vi "MixingGUI.vi"() -> ()   [LabVIEW 2016]
uses:
  <vilib>/Utility/miscctls.llb/LVStringsAndValuesArrayTypeDef.ctl
  <userlib>/Fluigent/Fluigent MFCS/FluigentMFCS_Full.llb/MFCS_EZ Detect.vi
  <userlib>/Fluigent/Fluigent MFCS/FluigentMFCS_Full.llb/MFCS_EZ Initialization.vi
  Labjack/ValveGlobals.vi
  Globals/PressuresGlobal.vi
  <vilib>/Utility/file.llb/Write Delimited Spreadsheet (string).vi
  <vilib>/Utility/file.llb/Read Delimited Spreadsheet (string).vi
  <userlib>/Fluigent/Fluigent MFCS/FluigentMFCS_Full.llb/MFCS_EZ Write Channel Pressure.vi
  <userlib>/_OpenG.lib/array/array.llb/Remove Duplicates from 1D Array (U16)__ogtk.vi
  <userlib>/Fluigent/Fluigent MFCS/FluigentMFCS_Full.llb/MFCS_EZ Close.vi
  <vilib>/MakerHub/Toolbox/LMH-Toolbox.lvlib
panel:
  out "Calibration Refs":T1
  out "Master Pressure Groups":u8[](array[numeric])=[3, 3, 3, 3, 4, 4, 4, 4, 2, 2]
  in  "Master Valves":u16(ring) items=["A1", "A2", "A3", "A4", "B1", "B2", "B3", "B4", "B5", "B6", "B7", "B8", "A5"]
  out "Set Pressures":dbl[][](array[numeric])
  out "Ctr Pressure":dbl=292.8560256927093
  in  "stop":bool
  in  "Tab Control":enum32{"Page 1", "Page 2"}(tab)
  in  "Reset All Calibrations":bool
  in  "Save Odor Inf File":bool
  in  "_run":i16=101
  in  "Sync Camera Acquisition":bool=TRUE
  in  "Ctr Water Valve":u16(ring)=15 items=["A1", "A2", "A3", "A4", "B1", "B2", "B3", "B4", "B5", "B6", "B7", "B8", "A5", "A6", "A7", "A8"]
  in  "Begin Experiment":bool
  in  "Log File Name":path=path "E:/maggot images/Orco_GCaMP"
  in  "Set to default pressure":bool
  in  "Mix Water Valve":u16(ring)=12 items=["A1", "A2", "A3", "A4", "B1", "B2", "B3", "B4", "B5", "B6", "B7", "B8", "A5", "A6", "A7", "A8"]
  in  "Mix Cluster":T2={"Ratio"=[0.6, 0.5], "Mix 2"=[12, 9], "Mix 1"=[0, 1]} {"Mix 1" items=["A1"=0, "A2"=1, "A3"=2, "A4"=3, "A5"=12]; "Mix 2" items=["B5"=8, "B6"=9, "B7"=10, "B8"=11, "A5"=12]}
  out "Ctr Pressure Group":u8=1
  out "Water Mix Pressure Group":u8=2
  in  "Close All Valves":bool
  in  "Odor":u16[](array[ring])=[0, 0, 0, 0, 0, 0, 0, 0] items=["1-pentanol", "3-pentanol", "3-octanol", "2,5-dimethylthiazole", "Add new..."]
  in  "Concentration":u16[](array[ring])=[0, 0, 0, 0, 0, 0, 0, 1] items=["10^-5", "10^-6", "Add new..."]
  in  "Odor Inf Path":path=path "C:/Users/Public/Documents/National Instruments/Fluigent/OdorInf/Data/OdorInfFiles/JB_20171127.txt"
  in  "Append Changes To Odor Inf File":bool=TRUE
  in  "Valves":u16[](array[ring])=[0, 1, 2, 3, 8, 9, 10, 11] items=["A1", "A2", "A3", "A4", "B1", "B2", "B3", "B4", "B5", "B6", "B7", "B8"]
  out "Pressure Group":u8[](array[numeric])=[3, 3, 3, 3, 4, 4, 4, 4]
  in  "Odor Time":dbl[](array[numeric])=[10.0, 10.0]
  in  "Water Time":dbl[](array[numeric])=[10.0, 10.0]
  in  "Number of Periods":dbl=2.0
  in  "Start Water":dbl=6.0
  out "Experiment Time (Sec)":dbl=46.0
  in  "Calibrate Pressures":bool
  out "Duplicates!":bool
  in  "Zero Pressure":bool
  in  "Ctr Odor Valve":u16(ring)=14 items=["A1", "A2", "A3", "A4", "B1", "B2", "B3", "B4", "B5", "B6", "B7", "B8", "A5", "A6", "A7", "A8"]
  in  "Calibration Mode":T3(ring)=enum."Odors Only"
  out "Calibration Required":bool=TRUE
  in  "Refill!":bool[](array[boolean])=[FALSE, FALSE, FALSE, FALSE, FALSE, FALSE, FALSE, FALSE, FALSE, FALSE, FALSE]
  out "Odor \nLevel":T4={"Tank"=10.0, "Tank 2"=10.0, "Tank 3"=10.0, "Tank 4"=10.0, "Tank 5"=10.0, "Tank 6"=10.0, "Tank 7"=10.0, "Tank 8"=10.0, "Tank 9"=10.0, "Tank 10"=10.0, "Tank 11"=10.0} {"Tank 11" scale=0.0..10.0; "Tank 10" scale=0.0..10.0; "Tank 9" scale=0.0..10.0; "Tank 8" scale=0.0..10.0; "Tank 7" scale=0.0..10.0; "Tank 6" scale=0.0..10.0; "Tank 5" scale=0.0..10.0; "Tank 4" scale=0.0..10.0; "Tank 3" scale=0.0..10.0; "Tank 2" scale=0.0..10.0; "Tank" scale=0.0..10.0}
  in  "Mix Water Pressure Channel":u16=2
  in  "Control Pressure Channel":u16=1
  out "Current Pressure":dbl[](array[numeric])=[1.2623618841171265, 1.893542766571045, 0.0, 2.524723768234253]
  in  "Manual Set Pressures":dbl[](array[numeric])=[292.8560256927093, 929.8857946603396, 888.3091798855597, 854.075528379124]
  in  "Total Odor Flow":dbl=425.0
  in  "Total Flow Setpoint":dbl=531.25
  out "Flow Meter 1 (water flow)":cluster{"[0]":dbl, "[1]":dbl}(graph)={"[0]"=0.1724137931034483, "[1]"=0.0}
  out "Flow Meter 2 (total flow)":cluster{"[0]":dbl, "[1]":dbl}(graph)={"[0]"=0.1724137931034483, "[1]"=0.0}
  in  "Values to Display":dbl=400.0
  out "Default Pressures":dbl[](array[numeric])=[292.8560256927093, 929.8857946603396, 888.3091798855597, 854.075528379124]
  in  "Master Ratio":dbl[](array[numeric])=[0.6, 0.6]
  in  "Master Mix 2":u16[](array[ring])=[12, 9, 11, 12, 11, 4, 4, 4] items=["B1"=4, "B2"=5, "B3"=6, "B4"=7, "A5"=12]
  in  "Master Mix 1":u16[](array[ring])=[0, 1, 1, 0, 0, 0, 0, 0] items=["A1"=0, "A2"=1, "A3"=2, "A4"=3, "A5"=12]
  in  "Master Water Time":dbl[](array[numeric])=[10.0, 10.0, 10.0, 10.0, 10.0, 10.0, 10.0, 10.0]
  in  "Master Odor Time":dbl[](array[numeric])=[10.0, 10.0, 10.0, 10.0, 10.0, 10.0, 10.0, 10.0]
  out "A5 in Both!":bool
  out "Master Valves":T5=[{"String"="A1", "Value"=0.0}, {"String"="A2", "Value"=1.0}, {"String"="A3", "Value"=2.0}, {"String"="A4", "Value"=3.0}, {"String"="B1", "Value"=4.0}, {"String"="B2", "Value"=5.0}, {"String"="B3", "Value"=6.0}, {"String"="B4", "Value"=7.0}, {"String"="B5", "Value"=8.0}, {"String"="B6", "Value"=9.0}, {"String"="B7", "Value"=10.0}, {"String"="B8", "Value"=11.0}, {"String"="A5", "Value"=12.0}]
  # "log_"
  # ".txt"
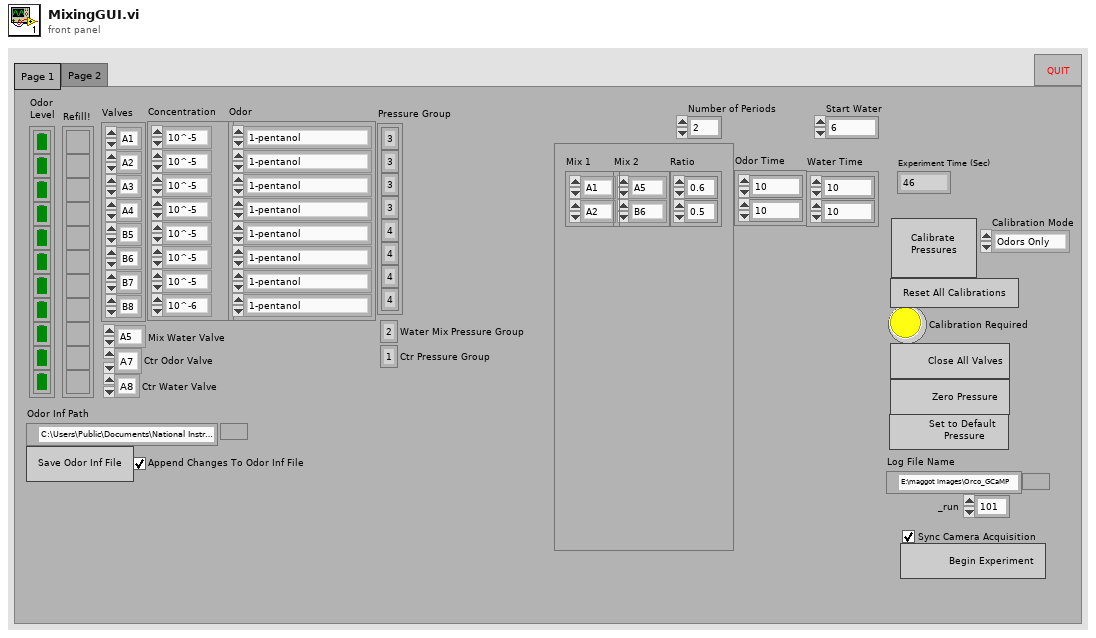
[diagram p1: front panel]
types:
  T1 = cluster{"Pressure Controller List":u8[], "Ratio List":dbl[], "Valve List":u16[]}
  T2 = cluster{"Ratio":dbl[], "Mix 2":u16[], "Mix 1":u16[]}
  T3 = enum16{"Calibrate All", "Control Only", "Odors Only"}
  T4 = cluster{"Tank":dbl, "Tank 2":dbl, "Tank 3":dbl, "Tank 4":dbl, "Tank 5":dbl, "Tank 6":dbl, "Tank 7":dbl, "Tank 8":dbl, "Tank 9":dbl, "Tank 10":dbl, "Tank 11":dbl}
  T5 = typedef "LVStringsAndValuesArrayTypeDef.ctl" = cluster{"String":string, "Value":ext}[]
  T6 = enum32{"Invalid", "Standard", "Closed", "Hidden", "Minimized", "Maximized"}
  T7 = cluster{"Ctr Odor Valve":u16, "Water Mix Valve":u16, "Total Odor Flow":dbl, "Total Flow Setpoint":dbl, "Control Pressure Channel":u16, "Mix Water Pressure Channel":u16}
  T8 = enum32{"Invalid", "Standard", "Closed", "Hidden", "Minimized", "Maximized"}[]
  T9 = typedef "_EZmfcsSN.ctl" = u16
  T10 = typedef "_EZmfcsRefNum.ctl" = refnum<k1>
  T11 = cluster{"[0]":dbl, "[1]":dbl, "[2]":dbl, "[3]":dbl, "[4]":dbl, "[5]":dbl, "[6]":dbl, "[7]":dbl, "[8]":dbl, "[9]":dbl, "[10]":dbl}
  T12 = cluster{"Flowboards":enum16{"A", "B", "C"}[], "Channels":enum16{"1", "2", "3", "4", "5", "6", "7", "8"}[], "States":bool[]}[]
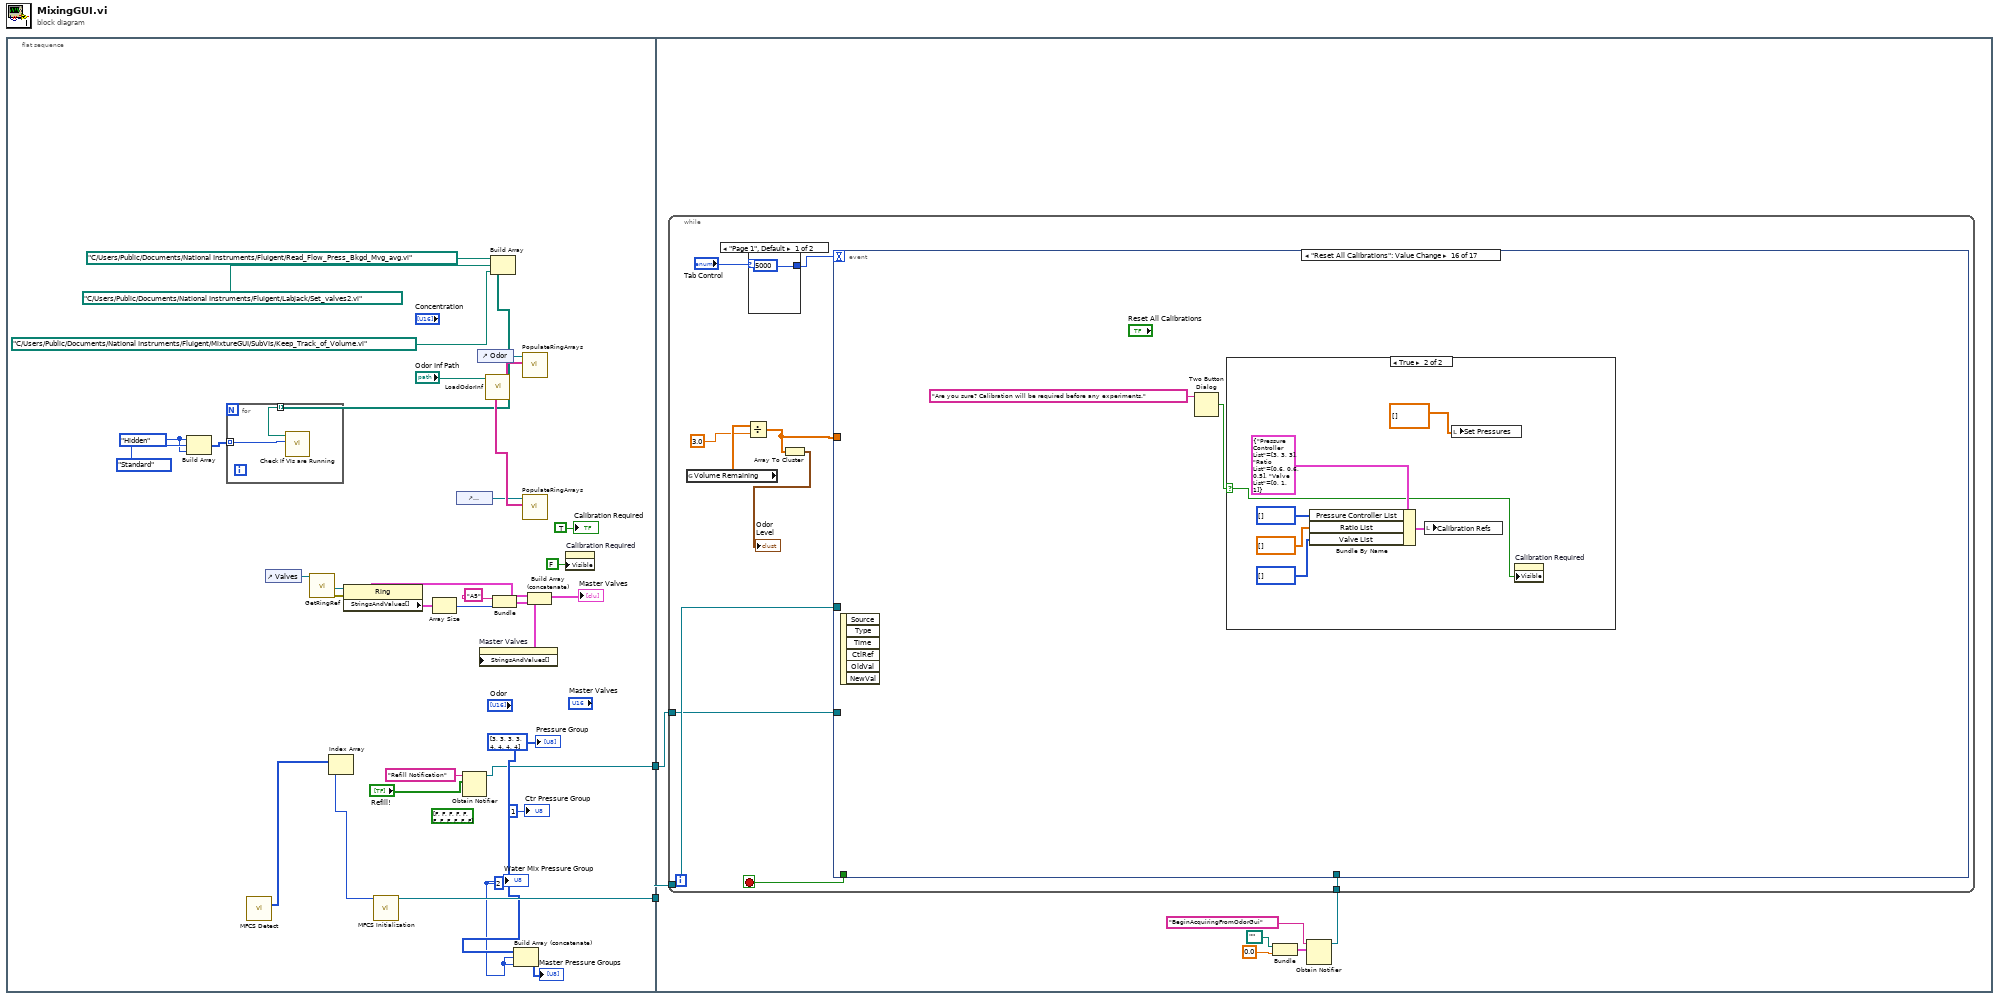
[diagram p0: block diagram]
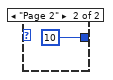
[diagram p2: hidden frame]
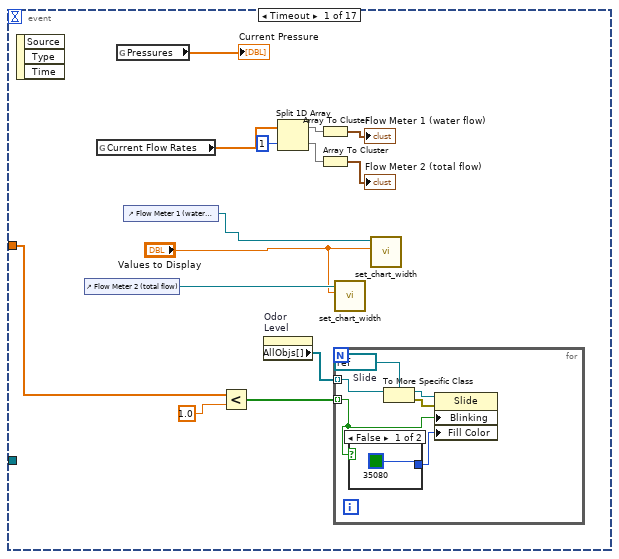
[diagram p3: hidden frame]
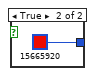
[diagram p4: hidden frame]
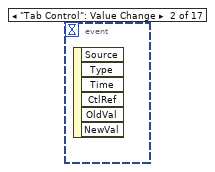
[diagram p5: hidden frame]
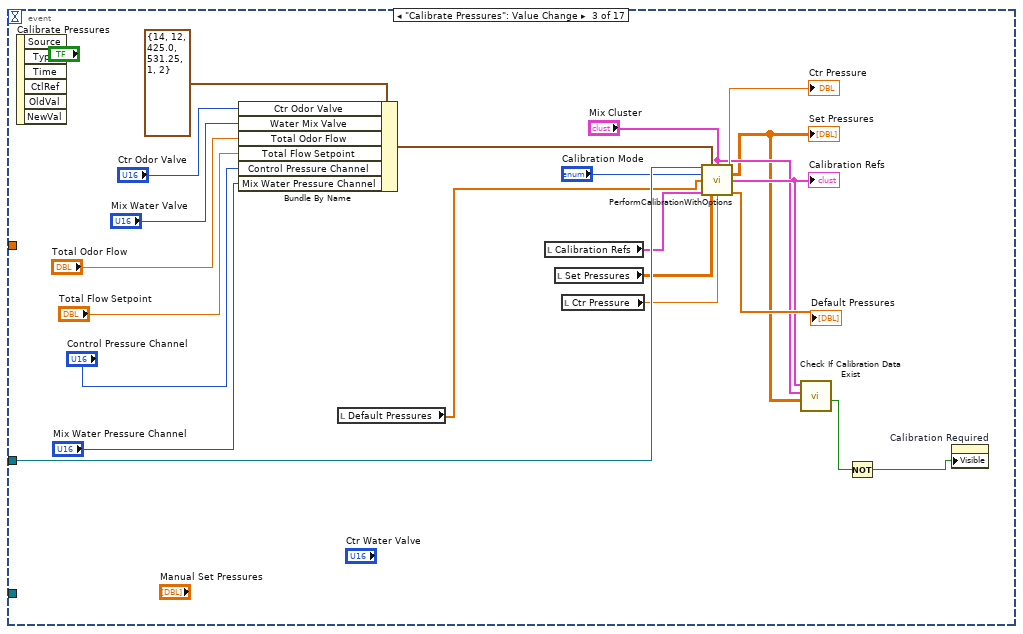
[diagram p6: hidden frame]
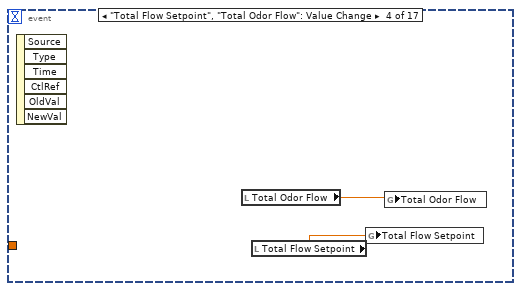
[diagram p7: hidden frame]
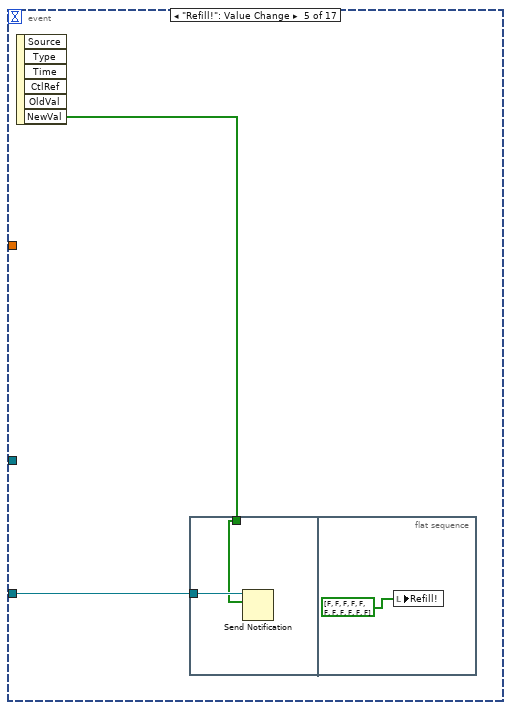
[diagram p8: hidden frame]
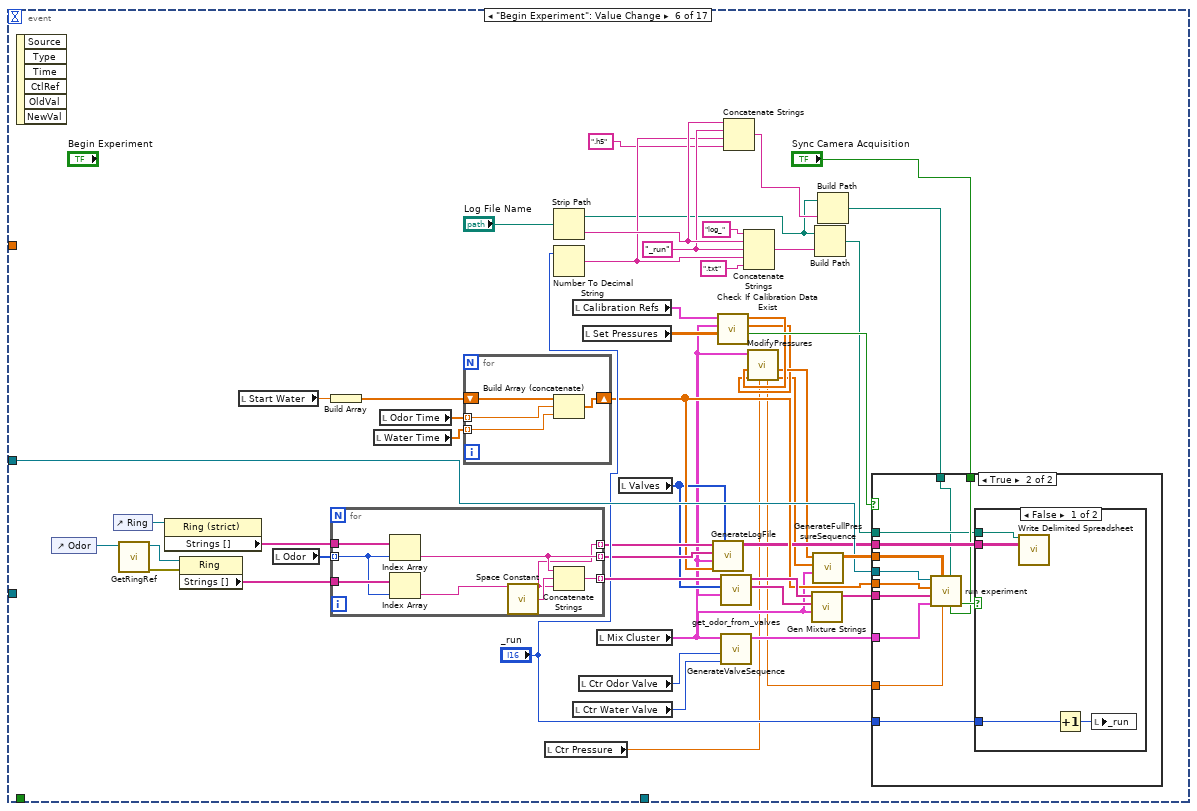
[diagram p9: hidden frame]
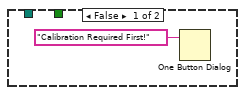
[diagram p10: hidden frame]
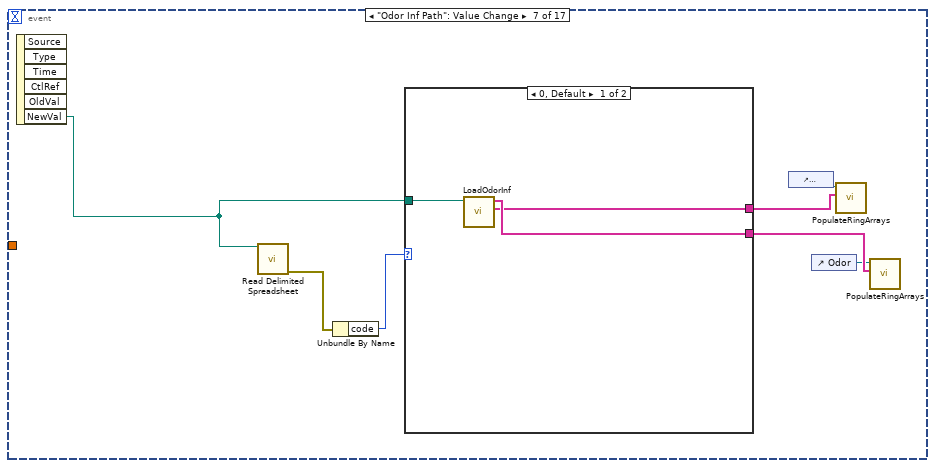
[diagram p12: hidden frame]
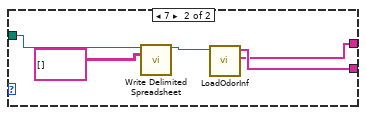
[diagram p13: hidden frame]
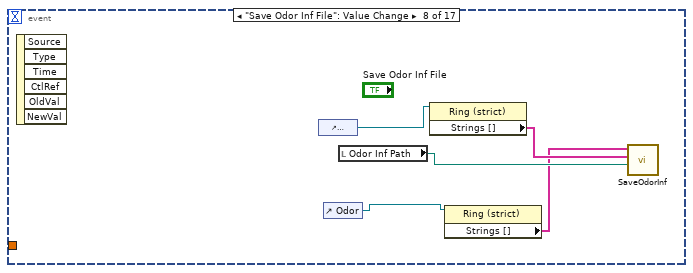
[diagram p14: hidden frame]
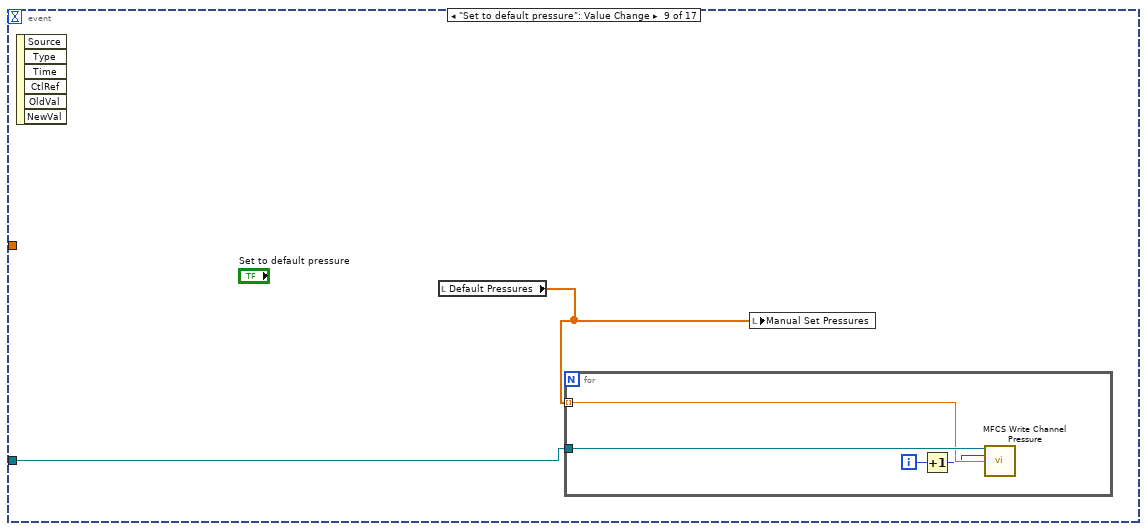
[diagram p15: hidden frame]
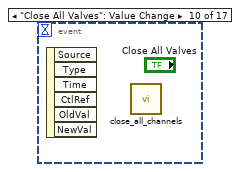
[diagram p16: hidden frame]
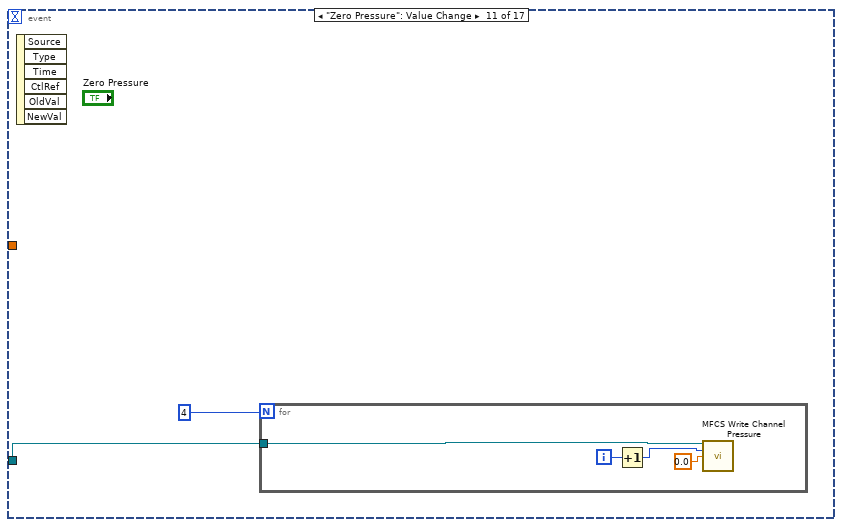
[diagram p17: hidden frame]
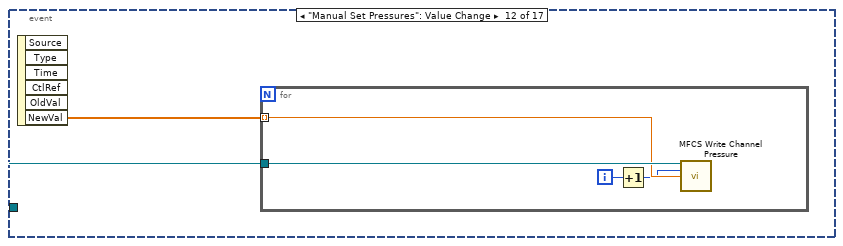
[diagram p18: hidden frame]
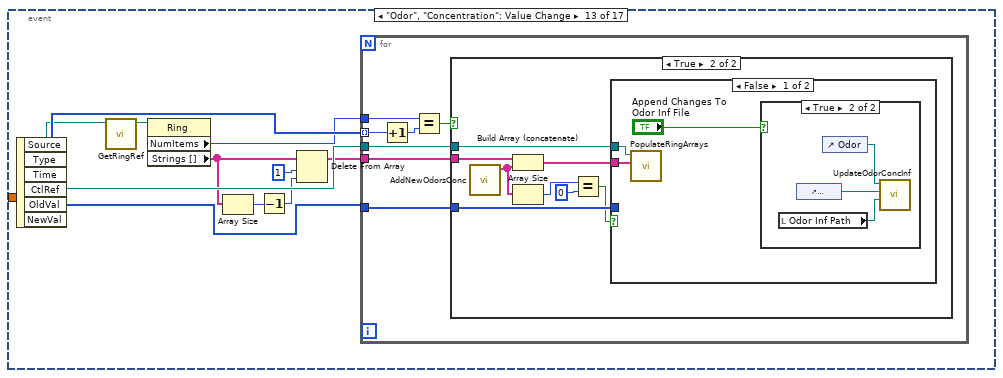
[diagram p19: hidden frame]
diagram:
  n1 = flat-sequence {
    tunnel: [w20] -> w2
    tunnel: [w6] -> w1
    tunnel: w2 -> [w43]
    tunnel: w1 -> [w37]
    frame #0 {
      (unwired) bool[] [FALSE, FALSE, FALSE, FALSE, FALSE, FALSE, FALSE, FALSE, FALSE, FALSE, FALSE] ("Refill!")
      w4 = T6."Hidden" ("State")
      w16 = u8 2 ("Water Mix Pressure Group")
      w18 = u8[] [3, 3, 3, 3, 4, 4, 4, 4] ("Pressure Group")
      n2 = Build Array(w4, T6."Standard" ("State"), w4) -> (w10:T8)
      n3 = call-poly <userlib>:"MFCS Detect.vi"() -> ("[SN MFCS_EZ]"=w22:T9[])  [unwired: 14 in, 1 out]
      n4 = control-ref of="Valves"() -> (w30:refnum<vi>)
      n5 = call "GetRingRef.vi"("Array Reference"=w30) -> ("error out"=w29:errorcluster, "Ring Reference"=w28:refnum<vi>)  [unwired: 9 in]
      n6 = Index Array(array=w22) -> (element=w21:T9)  [unwired: 1 in]
      n7 = property class="Ring"(reference=w28, error in=w29) -> ("StringsAndValues[]"=w34:T5)  [unwired: 2 out]
      n8 = call-poly <userlib>:"MFCS Initialization.vi"("SN MFCS_EZ"=w21) -> ("MFCS_EZ"=w20:T10)  [unwired: 12 in, 2 out]
      n9 = Array Size(array=w34) -> (size(s)=w32:i32)
      n10 = control-ref of="Concentration"() -> (w26:refnum<vi>)
      n11 = Obtain Notifier(name (unnamed)="Refill Notification", notification data type="Refill!") -> (notifier out=w6:refnum<notifier>)  [unwired: 2 in, 2 out]
      n12 = control-ref of="Odor"() -> (w24:refnum<vi>)
      n13 = call "LoadOdorInf.vi"("file path (dialog if empty)"="Odor Inf Path") -> ("Concentration"=w27:string[], "Odor"=w25:string[])  [unwired: 9 in]
      n14 = Build Array(path "C:/Users/Public/Documents/National Instruments/Fluigent/Read_Flow_Press_Bkgd_Mvg_avg.vi", path "C:/Users/Public/Documents/National Instruments/Fluigent/Labjack/Set_valves2.vi", path "C:/Users/Public/Documents/National Instruments/Fluigent/MixtureGUI/SubVIs/Keep_Track_of_Volume.vi") -> (w12:path[])
      n15 = for {
        tunnel: w12 -> [w36] mode=indexing
        tunnel: w10 -> [w35] mode=indexing
        n16 = call "Check If VIs are Running.vi"("State"=w35, "Path"=w36) -> ()  [unwired: 9 in, 1 out]
      }
      n17 = Bundle("A5", w32) -> (w33:cluster{string, i32})  [unwired: 1 in]
      n18 = Build Array (concatenate)(w18, w16, w16) -> (→"Master Pressure Groups":u8[])
      n19 = call "PopulateRingArrays.vi"("array"=w25, "Array Reference"=w24) -> ()  [unwired: 8 in, 2 out]
      n20 = call "PopulateRingArrays.vi"("array"=w27, "Array Reference"=w26) -> ()  [unwired: 8 in, 2 out]
      n21 = Build Array (concatenate)(w34, w33) -> (w19:T5)
      "Master Valves" <- w19
      n22 = property on="Master Valves" class="Ring (strict)"("StringsAndValues[]"=w19) -> ()  [unwired: 2 in, 2 out]
      n23 = property on="Calibration Required" class="Bool (strict)"("Visible"=FALSE) -> ()  [unwired: 2 in, 2 out]
      "Pressure Group" <- w18
      "Water Mix Pressure Group" <- w16
      "Ctr Pressure Group" <- u8 1 ("Ctr Pressure Group")
      "Calibration Required" <- TRUE ("Calibration Required")
    }
    frame #1 {
      n24 = Bundle("Log File Name"=path "", 0.0) -> (w39:cluster{"Log File Name":path, dbl})  [unwired: 1 in]
      n25 = Obtain Notifier(name (unnamed)="BeginAcquiringFromOdorGui", notification data type=w39) -> (notifier out=w41:refnum<notifier>)  [unwired: 2 in, 2 out]
      n26 = while {
        tunnel: w43 -> [w50]
        tunnel: w41 -> [w49]
        tunnel: w37 -> [w48]
        stop <- w53 stop-if-true
        n27 = global read "ValveGlobals.vi" "Volume Remaining"() -> (w47:dbl[])
        n28 = Divide(x=w47, y=3.0) -> (x/y=w44:dbl[])
        n29 = case shown="\"Page 1\", Default" "Tab Control" {
          tunnel: [5000 10] -> w51
          frame "Page 1", Default {
          }
          frame "Page 2" {
          }
        }
        n30 = Array To Cluster(array=w44) -> (cluster=→"Odor \nLevel":T11)
        n31 = event shown="[15] \"Reset All Calibrations\": Value Change" {
          selector: _ -> [_ _ _ _ _ _ _ _ _ _ _ _ _ _ _ _ _]
          dyn-events: _ -> [_ _ _ _ _ _ _ _ _ _ _ _ _ _ _ _ _]
          timeout: w51 -> [_ _ _ _ _ _ _ _ _ _ _ _ _ _ _ _ _]
          tunnel: [_ _ _ _ _ _ _ _ _ _ _ _ _ _ _ _ TRUE] -> w53
          tunnel: w50 -> [_ _ w98 _ _ w134 _ _ w203 _ w209 w216 _ _ _ _ w365]
          tunnel: w49 -> [_ _ _ _ _ _ _ _ _ _ _ _ _ _ _ _ _]
          tunnel: w48 -> [_ _ _ _ w102 _ _ _ _ _ _ _ _ _ _ _ _]
          tunnel: w44 -> [w56 _ _ _ _ _ _ _ _ _ _ _ _ _ _ _ _]
          event Timeout {
            n32 = event-data() -> ()  [unwired: 1 in, 3 out]
            n33 = control-ref of="Flow Meter 2 (total flow)"() -> (w61:refnum<vi>)
            n34 = global read "PressuresGlobal.vi" "Current Flow Rates"() -> (w66:dbl[])
            n35 = global read "PressuresGlobal.vi" "Pressures"() -> (→"Current Pressure":dbl[])
            n36 = control-ref of="Flow Meter 1 (water flow)"() -> (w62:refnum<vi>)
            n37 = Less?(x=w56, y=1.0) -> (x < y?=w58:bool[])
            n38 = property on="Odor \nLevel" class="Clust (strict)"() -> ("AllObjs[]"=w57:refnum<vi>[])  [unwired: 2 in, 2 out]
            n39 = Split 1D Array(array=w66, index=1) -> (first subarray=w64:dbl[], second subarray=w63:dbl[])
            n40 = Array To Cluster(array=w64) -> (cluster=→"Flow Meter 1 (water flow)":cluster{"[0]":dbl, "[1]":dbl})
            n41 = Array To Cluster(array=w63) -> (cluster=→"Flow Meter 2 (total flow)":cluster{"[0]":dbl, "[1]":dbl})
            n42 = for {
              tunnel: w58 -> [w71] mode=indexing
              tunnel: w57 -> [w75] mode=indexing
              w74 = refnum<vi> refnum  # Slide
              n43 = case shown="False" w71 {
                tunnel: [u32 35080 u32 15665920] -> w70
                frame False {
                }
                frame True {
                }
              }
              n44 = To More Specific Class(target class=w74, reference=w75) -> (specific class reference=w73:refnum<vi>, error out=w72:errorcluster)  [unwired: 1 in]
              n45 = property class="Slide"(reference=w73, error in=w72, "Blinking"=w71, "Fill Color"=w70) -> ()  [unwired: 2 out]
            }
            n46 = call "set_chart_width.vi"("Values to Display"="Values to Display", "Ctl Refnum"=w61) -> ()  [unwired: 10 in]
            n47 = call "set_chart_width.vi"("Values to Display"="Values to Display", "Ctl Refnum"=w62) -> ()  [unwired: 10 in]
          }
          event "Tab Control": Value Change {
            n48 = event-data() -> ()  [unwired: 1 in, 6 out]
          }
          event "Calibrate Pressures": Value Change {
            n49 = event-data() -> ()  [unwired: 1 in, 6 out]
            n50 = Bundle By Name(cluster=T7 {"Ctr Odor Valve"=14, "Water Mix Valve"=12, "Total Odor Flow"=425.0, "Total Flow Setpoint"=531.25, "Control Pressure Channel"=1, "Mix Water Pressure Channel"=2} ("Misselaneous Parameters"), "Ctr Odor Valve"="Ctr Odor Valve", "Water Mix Valve"="Mix Water Valve", "Total Odor Flow"="Total Odor Flow", "Total Flow Setpoint"="Total Flow Setpoint", "Control Pressure Channel"="Control Pressure Channel", "Mix Water Pressure Channel"="Mix Water Pressure Channel") -> (w92:T7)
            n51 = local read "Default Pressures"() -> (w83:dbl[])
            n52 = local read "Calibration Refs"() -> (w85:T1)
            n53 = local read "Set Pressures"() -> (w95:dbl[][])
            n54 = local read "Ctr Pressure"() -> (w94:dbl)
            n55 = call "PerformCalibrationWithOptions.vi"("MFCS_EZ"=w98, "Misselaneous Parameters"=w92, "Mix Cluster"="Mix Cluster", "Calibration Mode"="Calibration Mode", "Manual Default Set Pressures"=w83, "Calibration Refs In"=w85, "Set Pressures In"=w95, "Ctr Pressure In"=w94) -> ("Ctr Pressure Out"=→"Ctr Pressure":dbl, "Set Pressures Out"=w80:dbl[][], "Calibration Refs Out"=w82:T1, "Manual Default Set Pressures Out"=→"Default Pressures":dbl[])  [unwired: 3 in, 1 out]
            "Set Pressures" <- w80
            "Calibration Refs" <- w82
            n56 = call "Check If Calibration Data Exist.vi"("Set Pressures List"=w80, "Mix Cluster"="Mix Cluster", "Calibration Refs"=w82) -> ("Calibration Data Exists?"=w79:bool)  [unwired: 6 in, 2 out]
            n57 = Not(x=w79) -> (.not. x?=w78:bool)
            n58 = property on="Calibration Required" class="Bool (strict)"("Visible"=w78) -> ()  [unwired: 2 in, 2 out]
          }
          event "Total Flow Setpoint", "Total Odor Flow": Value Change {
            n59 = event-data() -> ()  [unwired: 1 in, 6 out]
            n60 = local read "Total Odor Flow"() -> (w100:dbl)
            n61 = local read "Total Flow Setpoint"() -> (w99:dbl)
            n62 = global write "ValveGlobals.vi" "Total Flow Setpoint"(w99) -> ()
            n63 = global write "ValveGlobals.vi" "Total Odor Flow"(w100) -> ()
          }
          event "Refill!": Value Change {
            n64 = event-data() -> ("NewVal"=w101:bool[])  [unwired: 1 in, 5 out]
            n65 = flat-sequence {
              tunnel: w102 -> [w104]
              tunnel: w101 -> [w103]
              frame #0 {
                n66 = Send Notification(notification=w103, notifier=w104) -> ()  [unwired: 1 in, 2 out]
              }
              frame #1 {
                n67 = local write "Refill!"(bool[] [FALSE, FALSE, FALSE, FALSE, FALSE, FALSE, FALSE, FALSE, FALSE, FALSE, FALSE] ("Refill!")) -> ()
              }
            }
          }
          event "Begin Experiment": Value Change {
            w111 = "_run" ("string")
            n68 = event-data() -> ()  [unwired: 1 in, 6 out]
            n69 = control-ref of="Odor"() -> (w151:refnum<vi>)
            n70 = control-ref of="Ring"() -> (w129:refnum<vi>)
            n71 = call "GetRingRef.vi"("Array Reference"=w151) -> ("error out"=w149:errorcluster, "Ring Reference"=w150:refnum<vi>)  [unwired: 9 in]
            n72 = property class="Ring (strict)"(reference=w129) -> ("Strings []"=w128:string[])  [unwired: 1 in, 2 out]
            n73 = property class="Ring"(reference=w150, error in=w149) -> ("Strings []"=w147:string[])  [unwired: 2 out]
            n74 = local read "Start Water"() -> (w142:dbl)
            n75 = local read "Odor"() -> (w148:u16[])
            n76 = Build Array(w142) -> (w141:dbl[])
            n77 = for {
              tunnel: w148 -> [w163] mode=indexing
              tunnel: w147 -> [w165]
              tunnel: [w161] -> w146 mode=indexing
              tunnel: w128 -> [w164]
              tunnel: [w160] -> w126 mode=indexing
              tunnel: [w159] -> w127 mode=indexing
              n78 = Index Array(array=w164, index=w163) -> (element=w160:string)
              n79 = Index Array(array=w165, index=w163) -> (element=w159:string)
              n80 = call <vilib>:"Space Constant.vi"() -> ("String"=w162:string)
              n81 = Concatenate Strings(w160, w162, w159) -> (w161:string)
            }
            n82 = local read "Water Time"() -> (w139:dbl[])
            n83 = local read "Odor Time"() -> (w140:dbl[])
            n84 = for {
              shift-right: [w155] -> w125
              shift-left: w141 -> [w157]
              tunnel: w140 -> [w158] mode=indexing
              tunnel: w139 -> [w156] mode=indexing
              n85 = Build Array (concatenate)(w157, w158, w156) -> (w155:dbl[])
            }
            n86 = local read "Ctr Pressure"() -> (w116:dbl)
            n87 = Strip Path(path="Log File Name") -> (stripped path=w107:path, name=w112:string)
            n88 = Number To Decimal String(number="_run") -> (decimal integer string=w110:string)  [unwired: 1 in]
            n89 = local read "Calibration Refs"() -> (w154:T1)
            n90 = local read "Ctr Water Valve"() -> (w144:u16)
            n91 = local read "Ctr Odor Valve"() -> (w145:u16)
            n92 = local read "Set Pressures"() -> (w153:dbl[][])
            n93 = local read "Mix Cluster"() -> (w117:T2)
            n94 = local read "Valves"() -> (w124:u16[])
            n95 = call "GenerateLogFile.vi"("Valves"=w124, "Sequence Time"=w125, "Mix Cluster"=w117, "Concentration Names"=w126, "Odor Names"=w127) -> ("LogFile"=w122:string[][])  [unwired: 6 in]
            n96 = call "Check If Calibration Data Exist.vi"("Set Pressures List"=w153, "Mix Cluster"=w117, "Calibration Refs"=w154) -> ("Calibration Data Exists?"=w152:bool, "Pressure For Mix 2"=w119:dbl[], "Pressure For Mix 1"=w121:dbl[])  [unwired: 6 in]
            n97 = call "get_odor_from_valves.vi"("Mix Cluster"=w117, "Valves"=w124, "Odor Names"=w146) -> ("Mix 2 Odors"=w138:string[], "Mix 1 Odors"=w137:string[])  [unwired: 7 in]
            n98 = call "GenerateValveSequence.vi"("Ctr Water Valve"=w144, "Ctr Odor Valve"=w145, "Mix Cluster"=w117) -> ("Valve Sequence Data"=w143:T12)  [unwired: 6 in, 2 out]
            n99 = Concatenate Strings(w112, w111, w110, ".h5" ("string")) -> (w108:string)
            n100 = Concatenate Strings("log_" ("string"), w112, w111, w110, ".txt" ("string")) -> (w131:string)
            n101 = call "ModifyPressures.vi"("Ctr Pressure In"=w116, "Pressure For Mix 2"=w119, "Pressure For Mix 1"=w121, "Mix Cluster"=w117) -> ("Modified Pressure for Mix 2"=w118:dbl[], "Modified Pressure for Mix 1"=w120:dbl[], "Control Pressure Out"=w115:dbl)  [unwired: 5 in]
            n102 = call "Gen Mixture Strings.vi"("Mix Cluster"=w117, "Mix 2 Odors"=w138, "Mix 1 Odors"=w137) -> ("mixture sequence array"=w136:string[])  [unwired: 7 in, 1 out]
            n103 = call "GenerateFullPressureSequence.vi"("Mix Cluster"=w117, "Pressure For Mix 2"=w118, "Pressure For Mix 1"=w120) -> ("Pressure Sequence (Ch 2-4)"=w135:dbl[][])  [unwired: 8 in]
            n104 = Build Path(base path=w107, name or relative path=w131) -> (appended path=w123:path)
            n105 = Build Path(base path=w107, name or relative path=w108) -> (appended path=w106:path)
            n106 = case shown="True" w152 {
              tunnel: w143 -> [_ w174]
              tunnel: w125 -> [_ w176]
              tunnel: w136 -> [_ w178]
              tunnel: w135 -> [_ w175]
              tunnel: w134 -> [_ w177]
              tunnel: w115 -> [_ w171]
              tunnel: "_run" -> [_ w172]
              tunnel: w123 -> [_ w168]
              tunnel: w122 -> [_ w170]
              tunnel: "Sync Camera Acquisition" -> [_ w169]
              tunnel: w106 -> [_ w167]
              frame False {
                n107 = One Button Dialog(message="Calibration Required First!") -> ()  [unwired: 1 in, 1 out]
              }
              frame True {
                n108 = call "run experiment.vi"("Sync Camera Acquisition"=w169, "Log File Name"=w167, "Ctr Odor Pressure"=w171, "Pressure Sequence (Ch 2-4)"=w175, "Valve Sequence Data"=w174, "mixture sequence array"=w178, "Time Sequence"=w176, "MFCS_EZ"=w177) -> ("Aborted?"=w173:bool)  [unwired: 3 in]
                n109 = case shown="False" w173 {
                  tunnel: w172 -> [w182 _]
                  tunnel: w168 -> [w180 _]
                  tunnel: w170 -> [w179 _]
                  frame False {
                    n110 = call-poly <vilib>:"Write Delimited Spreadsheet.vi"("file path (dialog if empty)"=w180, "2D data"=w179) -> ()  [unwired: 12 in, 2 out]
                    n111 = Increment(x=w182) -> (x+1=w181:i16)
                    n112 = local write "_run"(w181) -> ()
                  }
                  frame True {
                  }
                }
              }
            }
          }
          event "Odor Inf Path": Value Change {
            n113 = event-data() -> ("NewVal"=w187:path)  [unwired: 1 in, 5 out]
            n114 = call-poly <vilib>:"Read Delimited Spreadsheet.vi"("file path (dialog if empty)"=w187) -> ("error out"=w189:errorcluster)  [unwired: 9 in, 5 out]
            n115 = Unbundle By Name(w189) -> ("code"=w188:i32)
            n116 = case shown="0, Default" w188 {
              tunnel: w187 -> [w192 w197]
              tunnel: [w191 w194] -> w186
              tunnel: [w190 w193] -> w185
              frame 0, Default {
                n117 = call "LoadOdorInf.vi"("file path (dialog if empty)"=w192) -> ("Concentration"=w190:string[], "Odor"=w191:string[])  [unwired: 9 in]
              }
              frame 7 {
                n118 = call-poly <vilib>:"Write Delimited Spreadsheet.vi"("file path (dialog if empty)"=w197, "2D data"=string[][] []) -> ("new file path (Not A Path if cancelled)"=w195:path)  [unwired: 12 in, 1 out]
                n119 = call "LoadOdorInf.vi"("file path (dialog if empty)"=w195) -> ("Concentration"=w193:string[], "Odor"=w194:string[])  [unwired: 9 in]
              }
            }
            n120 = control-ref of="Concentration"() -> (w184:refnum<vi>)
            n121 = control-ref of="Odor"() -> (w183:refnum<vi>)
            n122 = call "PopulateRingArrays.vi"("array"=w185, "Array Reference"=w184) -> ()  [unwired: 8 in, 2 out]
            n123 = call "PopulateRingArrays.vi"("array"=w186, "Array Reference"=w183) -> ()  [unwired: 8 in, 2 out]
          }
          event "Save Odor Inf File": Value Change {
            n124 = event-data() -> ()  [unwired: 1 in, 6 out]
            n125 = control-ref of="Concentration"() -> (w200:refnum<vi>)
            n126 = control-ref of="Odor"() -> (w199:refnum<vi>)
            n127 = local read "Odor Inf Path"() -> (w202:path)
            n128 = property class="Ring (strict)"(reference=w200) -> ("Strings []"=w201:string[])  [unwired: 1 in, 2 out]
            n129 = property class="Ring (strict)"(reference=w199) -> ("Strings []"=w198:string[])  [unwired: 1 in, 2 out]
            n130 = call "SaveOdorInf.vi"("Path"=w202, "Concentrations"=w201, "Odors"=w198) -> ()  [unwired: 9 in]
          }
          event "Set to default pressure": Value Change {
            n131 = event-data() -> ()  [unwired: 1 in, 6 out]
            n132 = local read "Default Pressures"() -> (w204:dbl[])
            n133 = for {
              tunnel: w203 -> [w208]
              tunnel: w204 -> [w207] mode=indexing
              i -> [w206]
              n134 = Increment(x=w206) -> (x+1=w205:i32)
              n135 = call-poly <userlib>:"MFCS Write Channel Pressure.vi"("MFCS_EZ"=w208, "Channel Number (default=1)"=w205, "Pressure (mBar)"=w207) -> ()  [unwired: 11 in, 2 out]
            }
            n136 = local write "Manual Set Pressures"(w204) -> ()
          }
          event "Close All Valves": Value Change {
            n137 = event-data() -> ()  [unwired: 1 in, 6 out]
            n138 = call "close_all_channels.vi"() -> ()  [unwired: 12 in]
          }
          event "Zero Pressure": Value Change {
            n139 = event-data() -> ()  [unwired: 1 in, 6 out]
            n140 = for {
              N: 4 -> [_]
              tunnel: w209 -> [w211]
              i -> [w214]
              n141 = Increment(x=w214) -> (x+1=w213:i32)
              n142 = call-poly <userlib>:"MFCS Write Channel Pressure.vi"("MFCS_EZ"=w211, "Channel Number (default=1)"=w213, "Pressure (mBar)"=0.0) -> ()  [unwired: 11 in, 2 out]
            }
          }
          event "Manual Set Pressures": Value Change {
            n143 = event-data() -> ("NewVal"=w215:dbl[])  [unwired: 1 in, 5 out]
            n144 = for {
              tunnel: w216 -> [w220]
              tunnel: w215 -> [w219] mode=indexing
              i -> [w218]
              n145 = Increment(x=w218) -> (x+1=w217:i32)
              n146 = call-poly <userlib>:"MFCS Write Channel Pressure.vi"("MFCS_EZ"=w220, "Channel Number (default=1)"=w217, "Pressure (mBar)"=w219) -> ()  [unwired: 11 in, 2 out]
            }
          }
          event "Odor", "Concentration": Value Change {
            n147 = event-data() -> ("CtlRef"=w227:refnum<vi>, "OldVal"=w221:u16[], "NewVal"=w229:u16[])  [unwired: 1 in, 3 out]
            n148 = call "GetRingRef.vi"("Array Reference"=w227) -> ("Ring Reference"=w230:refnum<vi>)  [unwired: 9 in, 1 out]
            n149 = property class="Ring"(reference=w230) -> ("NumItems"=w228:u32, "Strings []"=w226:string[])  [unwired: 1 in, 2 out]
            n150 = Array Size(array=w226) -> (size(s)=w225:i32)
            n151 = Decrement(x=w225) -> (x-1=w222:i32)
            n152 = Delete From Array(array=w226, length=1, index=w222) -> (array with subset deleted=w223:string[])  [unwired: 1 out]
            n153 = for {
              tunnel: w229 -> [w237] mode=indexing
              tunnel: w228 -> [w236]
              tunnel: w227 -> [w234]
              tunnel: w223 -> [w233]
              tunnel: w221 -> [w231]
              n154 = Increment(x=w237) -> (x+1=w232:u16)
              n155 = Equal?(x=w236, y=w232) -> (x = y?=w235:bool)
              n156 = case shown="True" w235 {
                tunnel: w234 -> [_ w244]
                tunnel: w233 -> [_ w245]
                tunnel: w231 -> [_ w243]
                frame False {
                }
                frame True {
                  n157 = call "AddNewOdorsConc.vi"() -> ("To Add Out"=w241:string[])  [unwired: 10 in]
                  n158 = Build Array (concatenate)(w245, w241) -> (w242:string[])
                  n159 = Array Size(array=w241) -> (size(s)=w240:i32)
                  n160 = Equal?(x=w240, y=0 ("size(s)")) -> (x = y?=w238:bool)
                  n161 = case shown="False" w238 {
                    tunnel: w244 -> [w248 w253]
                    tunnel: w243 -> [_ w252]
                    tunnel: w242 -> [w247 _]
                    frame False {
                      n162 = call "PopulateRingArrays.vi"("array"=w247, "Array Reference"=w248) -> ()  [unwired: 8 in, 2 out]
                      n163 = case shown="True" "Append Changes To Odor Inf File" {
                        frame False {
                        }
                        frame True {
                          n164 = local read "Odor Inf Path"() -> (w249:path)
                          n165 = control-ref of="Concentration"() -> (w251:refnum<vi>)
                          n166 = control-ref of="Odor"() -> (w250:refnum<vi>)
                          n167 = call "UpdateOdorConcInf.vi"("Path"=w249, "Concentration Ref"=w251, "Odor Ref"=w250) -> ()  [unwired: 9 in]
                        }
                      }
                    }
                    frame True {
                      n168 = property class="Arr (strict)"(reference=w253, "Value"=w252) -> ()  [unwired: 1 in, 2 out]
                    }
                  }
                }
              }
            }
          }
          event "Valves": Value Change {
            # "greater than 0 means there are duplicates"
            n169 = event-data() -> ("NewVal"=w257:u16[])  [unwired: 1 in, 5 out]
            n170 = call-poly <userlib>:"Remove Duplicates from 1D Array__ogtk.vi"("Input Array"=w257) -> ("indices of removed elements"=w261:i32[])  [unwired: 1 out]
            n171 = local read "Ctr Water Valve"() -> (w254:u16)
            n172 = local read "Ctr Odor Valve"() -> (w255:u16)
            n173 = Array Size(array=w261) -> (size(s)=w259:i32)
            n174 = Greater?(x=w259, y=0 ("x")) -> (0:w258:bool)
            "Duplicates!" <- w258
            n175 = property on="Duplicates!" class="Bool (strict)"("Blinking"=w258, "Visible"=w258) -> ()  [unwired: 2 in, 2 out]
            n176 = global write "ValveGlobals.vi" "Ctr Odor Valve"(w255) -> ()
            n177 = global write "ValveGlobals.vi" "Ctr Water Valve"(w254) -> ()
            n178 = global write "ValveGlobals.vi" "Valves Used"("Valves") -> ()
            n179 = case shown="False" w258 {
              tunnel: w257 -> [w275 _]
              frame False {
                w289 = 4 ("index")
                n180 = control-ref of="Valves"() -> (w292:refnum<vi>)
                n181 = call "GetRingRef.vi"("Array Reference"=w292) -> ("error out"=w290:errorcluster, "Ring Reference"=w291:refnum<vi>)  [unwired: 9 in]
                n182 = property class="Ring"(reference=w291, error in=w290) -> ("StringsAndValues[]"=w265:T5)  [unwired: 2 out]
                n183 = local read "Mix Cluster"() -> (w263:T2)
                n184 = for {
                  tunnel: w275 -> [w294] mode=indexing
                  tunnel: w265 -> [w295]
                  tunnel: [w293] -> w278 mode=indexing
                  n185 = Index Array(array=w295, index=w294) -> (element=w293:cluster{"String":string, "Value":ext})
                }
                n186 = Array Size(array=w265) -> (size(s)=w264:i32)
                n187 = Unbundle By Name(w263) -> ("Mix 1"=w262:u16[])
                n188 = Split 1D Array(array=w275, index=w289) -> (first subarray=w271:u16[], second subarray=w272:u16[])
                n189 = Array Size(array=w262) -> (size(s)=w268:i32)
                n190 = Index Array(array=w271, index=0) -> (element=w270:u16)
                n191 = Index Array(array=w272, index=0) -> (element=w269:u16)
                n192 = Bundle("A5", w264) -> (w287:cluster{string, i32})  [unwired: 1 in]
                n193 = control-ref of="Mix 1"() -> (w276:refnum<vi>)
                n194 = control-ref of="Mix 2"() -> (w277:refnum<vi>)
                n195 = Initialize Array(w270, w268) -> (w267:u16[])
                n196 = Initialize Array(w269, w268) -> (w266:u16[])
                n197 = Split 1D Array(array=w278, index=w289) -> (first subarray=w285:cluster{"String":string, "Value":ext}[], second subarray=w286:cluster{"String":string, "Value":ext}[])
                n198 = property class="Arr (strict)"(reference=w276, "Value"=w267) -> ()  [unwired: 1 in, 2 out]
                n199 = call "GetRingRef.vi"("Array Reference"=w276) -> ("error out"=w283:errorcluster, "Ring Reference"=w284:refnum<vi>)  [unwired: 9 in]
                n200 = Build Array (concatenate)(w285, w287) -> (w279:cluster{"String":string, "Value":ext}[])
                n201 = property class="Arr (strict)"(reference=w277, "Value"=w266) -> ()  [unwired: 1 in, 2 out]
                n202 = call "GetRingRef.vi"("Array Reference"=w277) -> ("error out"=w281:errorcluster, "Ring Reference"=w282:refnum<vi>)  [unwired: 9 in]
                n203 = Build Array (concatenate)(w286, w287) -> (w280:cluster{"String":string, "Value":ext}[])
                n204 = property class="Ring"(reference=w284, error in=w283, "StringsAndValues[]"=w279) -> ()  [unwired: 2 out]
                n205 = property class="Ring"(reference=w282, error in=w281, "StringsAndValues[]"=w280) -> ()  [unwired: 2 out]
              }
              frame True {
              }
            }
          }
          event "Number of Periods", "Mix Cluster.Mix 1", "Mix Cluster.Mix 2": Value Change {
            n206 = event-data() -> ()  [unwired: 1 in, 6 out]
            n207 = local read "Master Valves"() -> (w337:T5)
            n208 = local read "Mix Cluster"() -> (w309:T2)
            n209 = Array Size(array=w337) -> (size(s)=w327:i32)
            n210 = Unbundle By Name(w309) -> ("Mix 2"=w304:u16[], "Mix 1"=w303:u16[])  [unwired: 1 out]
            n211 = Decrement(x=w327) -> (x-1=w326:i32)
            n212 = Search 1D Array(1D array=w304, element=w326) -> (index of element=w336:i32)  [unwired: 1 in]
            n213 = Search 1D Array(1D array=w303, element=w326) -> (index of element=w333:i32)  [unwired: 1 in]
            n214 = control-ref of="Water Time"() -> (w345:refnum<vi>)
            n215 = control-ref of="Odor Time"() -> (w353:refnum<vi>)
            n216 = control-ref of="Mix 2"() -> (w339:refnum<vi>)
            n217 = control-ref of="Mix 1"() -> (w338:refnum<vi>)
            n218 = control-ref of="Ratio"() -> (w325:refnum<vi>)
            n219 = Add Array Elements(numeric array="Water Time") -> (sum=w318:dbl)
            n220 = Add Array Elements(numeric array="Odor Time") -> (sum=w317:dbl)
            n221 = call "MakeArrayRightSize.vi"("Size"="Number of Periods", "Master Array In"="Master Water Time", "Array"="Water Time", "reference"=w345) -> ("Array Out"=w346:variant[], "Master Array Out"=w347:variant[])  [unwired: 6 in]
            n222 = call "MakeArrayRightSize.vi"("Size"="Number of Periods", "Master Array In"="Master Mix 2", "Array"=w304, "reference"=w339) -> ("Array Out"=w312:variant[], "Master Array Out"=w311:variant[])  [unwired: 6 in]
            n223 = call "MakeArrayRightSize.vi"("Size"="Number of Periods", "Master Array In"="Master Mix 1", "Array"=w303, "reference"=w338) -> ("Array Out"=w308:variant[], "Master Array Out"=w307:variant[])  [unwired: 6 in]
            n224 = call "MakeArrayRightSize.vi"("Size"="Number of Periods", "Master Array In"="Master Odor Time", "Array"="Odor Time", "reference"=w353) -> ("Array Out"=w351:variant[], "Master Array Out"=w349:variant[])  [unwired: 6 in]
            n225 = Equal?(x=w336, y=-1) -> (x = y?=w332:bool)
            n226 = Equal?(x=w333, y=-1) -> (x = y?=w331:bool)
            n227 = call "MakeArrayRightSize.vi"("Size"="Number of Periods", "Master Array In"="Master Ratio", "reference"=w325) -> ("Array Out"=w323:variant[], "Master Array Out"=w324:variant[])  [unwired: 7 in]
            n228 = Add(x=w318, y=w317) -> (x+y=w316:dbl)
            n229 = Variant To Data(type="Water Time", Variant=w347) -> (data=w342:dbl[])  [unwired: 1 in, 1 out]
            n230 = Variant To Data(type="Water Time", Variant=w346) -> (data=w343:dbl[])  [unwired: 1 in, 1 out]
            n231 = Variant To Data(type=w304, Variant=w312) -> (data=w313:u16[])  [unwired: 1 in, 1 out]
            n232 = Variant To Data(type=w303, Variant=w308) -> (data=w301:u16[])  [unwired: 1 in, 1 out]
            n233 = Variant To Data(type="Master Ratio", Variant=w324) -> (data=w302:dbl[])  [unwired: 1 in, 1 out]
            n234 = Variant To Data(type="Odor Time", Variant=w349) -> (data=w348:dbl[])  [unwired: 1 in, 1 out]
            n235 = Variant To Data(type="Odor Time", Variant=w351) -> (data=w350:dbl[])  [unwired: 1 in, 1 out]
            n236 = Variant To Data(Variant=w311) -> (data=w310:u16[])  [unwired: 2 in, 1 out]
            n237 = Variant To Data(Variant=w307) -> (data=w306:u16[])  [unwired: 2 in, 1 out]
            n238 = Variant To Data(Variant=w323) -> (data=w322:dbl[])  [unwired: 2 in, 1 out]
            n239 = Not(x=w332) -> (.not. x?=w328:bool)
            n240 = Not(x=w331) -> (.not. x?=w329:bool)
            n241 = local write "Master Water Time"(w342) -> ()
            n242 = local write "Water Time"(w343) -> ()
            n243 = local write "Master Mix 2"(w310) -> ()
            n244 = local write "Master Mix 1"(w306) -> ()
            n245 = local write "Master Ratio"(w322) -> ()
            n246 = local write "Master Odor Time"(w348) -> ()
            n247 = local write "Odor Time"(w350) -> ()
            n248 = Bundle By Name(cluster=w309, "Ratio"=w302, "Mix 2"=w313, "Mix 1"=w301) -> (w299:T2)
            n249 = And(x=w328, y=w329) -> (x .and. y?=w330:bool)
            "A5 in Both!" <- w330
            n250 = local read "Calibration Refs"() -> (w300:T1)
            n251 = local write "Mix Cluster"(w299) -> ()
            n252 = property on="A5 in Both!" class="Bool (strict)"("Visible"=w330, "Blinking"=w330) -> ()  [unwired: 2 in, 2 out]
            n253 = Add(x="Start Water", y=w316) -> (x+y=→"Experiment Time (Sec)":dbl)
            n254 = local read "Set Pressures"() -> (w298:dbl[][])
            n255 = call "Check If Calibration Data Exist.vi"("Set Pressures List"=w298, "Mix Cluster"=w299, "Calibration Refs"=w300) -> ("Calibration Data Exists?"=w297:bool)  [unwired: 6 in, 2 out]
            n256 = Not(x=w297) -> (.not. x?=w296:bool)
            n257 = property on="Calibration Required" class="Bool (strict)"("Visible"=w296) -> ()  [unwired: 2 in, 2 out]
          }
          event "Reset All Calibrations": Value Change {
            n258 = event-data() -> ()  [unwired: 1 in, 6 out]
            n259 = Two Button Dialog(message="Are you sure? Calibration will be required before any experiments.") -> (T button?=w354:bool)  [unwired: 2 in]
            n260 = case shown="True" w354 {
              selector: w354 -> [_ w356]
              frame False {
              }
              frame True {
                n261 = Bundle By Name(cluster=T1 {"Pressure Controller List"=[3, 3, 3], "Ratio List"=[0.6, 0.6, 0.5], "Valve List"=[0, 1, 1]} ("Calibration Refs"), "Pressure Controller List"=u8[] [], "Ratio List"=dbl[] [], "Valve List"=u16[] []) -> (w358:T1)
                n262 = local write "Calibration Refs"(w358) -> ()
                n263 = local write "Set Pressures"(dbl[][] []) -> ()
                n264 = property on="Calibration Required" class="Bool (strict)"("Visible"=w356) -> ()  [unwired: 2 in, 2 out]
              }
            }
          }
          event "stop": Value Change {
            n265 = event-data() -> ()  [unwired: 1 in, 6 out]
            n266 = call-poly <userlib>:"MFCS Close.vi"("MFCS_EZ"=w365) -> ()  [unwired: 14 in, 1 out]
            n267 = call "close_all_channels.vi"() -> ()  [unwired: 12 in]
            n268 = control-ref of="This VI"() -> (w363:refnum<vi>)
            n269 = call <vilib>:"Save State As Default.vi"("Target VI"=w363) -> ()  [unwired: 9 in, 2 out]
          }
        }
      }
    }
  }
